vi "SWERVE_MODULE_ACQUIRE.vi"(7 "MC type Drv":T1(ring), 8 "Drv Gear Ratio":dbl, 9 "Wheel Diameter IN":dbl=4.0 format="%#_13g", 10 "Encoder Name":string, 11 "Drive Motor Name":string) -> (0 "SWERVE_DRIVE_MODULE_POSITION":T2={"Distance"=0.0, "Angle"={"VALUE"=0.0, "COS"=1.0, "SIN"=0.0}, "P"=FALSE} {"Angle"."SIN" format="%13.4f"; "Angle"."COS" format="%13.4f"; "Angle"."VALUE" format="%13.4f"}, 2 "SWERVE_DRIVE_MODULE_STATE":T4={"Speed"=0.0, "Angle"={"VALUE"=0.0, "COS"=1.0, "SIN"=0.0}} {"Angle"."SIN" format="%13.4f"; "Angle"."COS" format="%13.4f"; "Angle"."VALUE" format="%13.4f"})   [LabVIEW 2023]
uses:
  <vilib>/Rock Robotics/WPI/ThirdParty/JAS_Junk/TrajLib/Trajectory_Library.lvlib
  <vilib>/Rock Robotics/WPI/ThirdParty/JAS_Junk/TrajLib/TypeDef/DCMOTOR.CTL
  <vilib>/Analysis/Matrix/Datatypes/RealMatrix.ctl
  <vilib>/Analysis/Matrix/NI_Matrix.lvlib
  <vilib>/Rock Robotics/WPI/ThirdParty/JAS_Junk/TrajLib/TypeDef/LINEAR_SYSTEM.ctl
  <vilib>/Rock Robotics/WPI/ThirdParty/JAS_Junk/TrajLib/TypeDef/LINEAR_SYSTEM_SIM.ctl
  <vilib>/Rock Robotics/WPI/ThirdParty/JAS_Junk/TrajLib/TypeDef/DCMOTOR_SIM.ctl
  <vilib>/Rock Robotics/Network Tables/NT Read Variant.vi
  SWERVE_DRIVE_GLOBALS.vi
  <vilib>/Rock Robotics/WPI/ThirdParty/Phoenix-LabVIEW/Motor Controller/Get/CTRE_Phoenix_MotorController_GetSelectedSensorData.vi
  <vilib>/Rock Robotics/WPI/ThirdParty/Phoenix-LabVIEW/CANCoder/Get/CTRE_Phoenix_CANcoder_GetSensorData.vi
  <vilib>/Rock Robotics/WPI/ThirdParty/REV Robotics/REVLib/SubVI/Public/SPARK Get Encoder Status Position.vi
  <vilib>/Rock Robotics/WPI/ThirdParty/Phoenix6/getters/GetPRO_PosAndVel_Velocity.vi
  <vilib>/Rock Robotics/WPI/ThirdParty/Phoenix6/getters/GetPRO_PosAndVel_Position.vi
  <vilib>/Rock Robotics/WPI/ThirdParty/REV Robotics/REVLib/SubVI/Public/SPARK Get Encoder Status Velocity.vi
  <vilib>/Rock Robotics/WPI/ThirdParty/JAS_Junk/TrajLib/TypeDef/ROTATION2D.ctl
  <vilib>/Rock Robotics/WPI/ThirdParty/JAS_Junk/TrajLib/TypeDef/SWERVE_DRIVE_MODULE_STATE.ctl
  <vilib>/Rock Robotics/WPI/ThirdParty/JAS_Junk/TrajLib/TypeDef/SWERVE_DRIVE_MODULE_POSITION.ctl
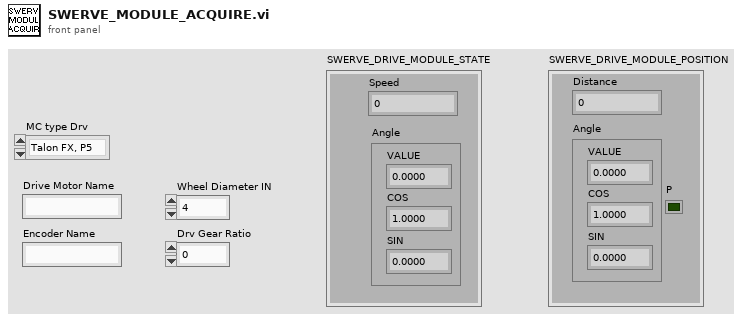
[diagram p1: front panel]
types:
  T1 = enum16{"Talon FX, P5", "Talon FX, P6", "SPARK MAX"}
  T2 = typedef "Trajectory_Library.lvlib/SWERVE_DRIVE_MODULE_POSITION.ctl" = cluster{"Distance":dbl, "Angle":T3, "P":bool}
  T3 = typedef "Trajectory_Library.lvlib/ROTATION2D.ctl" = cluster{"VALUE":dbl, "COS":dbl, "SIN":dbl}
  T4 = typedef "Trajectory_Library.lvlib/SWERVE_DRIVE_MODULE_STATE.ctl" = cluster{"Speed":dbl, "Angle":T3}
  T5 = typedef "Trajectory_Library.lvlib/DCMOTOR_SIM.ctl" = cluster{"LinearSystemSim":T6, "GearBox":T9, "Gearing":dbl}
  T6 = typedef "Trajectory_Library.lvlib/LINEAR_SYSTEM_SIM.ctl" = cluster{"m_Plant":T7, "m_X":T8, "m_Y":T8, "m_U":T8, "MeasureStdDev":T8}
  T7 = typedef "Trajectory_Library.lvlib/LINEAR_SYSTEM.ctl" = cluster{"m_A":T8, "m_B":T8, "m_C":T8, "m_D":T8, "States":i32, "Inputs":i32, "Outputs":i32}
  T8 = typedef "NI_Matrix.lvlib/RealMatrix.ctl" = dbl[][]
  T9 = typedef "Trajectory_Library.lvlib/DCMOTOR.CTL" = cluster{"nominalVoltage_Volts":dbl, "StallTorque_NM":dbl, "StallCurrent_Amps":dbl, "FreeCurrent_Amps":dbl, "FreeSpeed_RadPerSec":dbl, "R_Ohms":dbl, "KvINV_RadPerSecPerVolt":dbl, "Kt_NMPerAmp":dbl, "L_H":dbl, "Jr_KgM2":dbl}
  T10 = typedef "WPI_MotorControlDeviceRef.ctl" = cluster{"DeviceStatus":errorcluster, "Type":T11, "PWM":cluster{"PWM Channel":T12, "DeadBand":T13}, "CAN":cluster{"Device Number":u8, "SetOutput VI Ref":variant, "GetOutput VI Ref":variant, "Enable VI Ref":variant, "Disable VI Ref":variant, "Data":variant}, "Invert":bool, "DIO PWM":cluster{"PWM \"Enable\" Channel":T12, "DIOChannel":T14, "PWM Rate":dbl}}
  T11 = typedef "WPI_MotorControlType.ctl" = enum16{"PWM", "CAN", "DIO PWM"}
  T12 = typedef "FPGA_DIOPWMChannel.ctl" = enum8{"PWM 0", "PWM 1", "PWM 2", "PWM 3", "PWM 4", "PWM 5", "PWM 6", "PWM 7", "PWM 8", "PWM 9", "PWM MXP 0", "PWM MXP 1", "PWM MXP 2", "PWM MXP 3", "PWM MXP 4", "PWM MXP 5", "PWM MXP 6", "PWM MXP 7", "PWM MXP 8", "PWM MXP 9", "Invalid"}
  T13 = typedef "WPI_PWMDeadband.ctl" = cluster{"Name":string, "maxPositivePwm":i32, "minPositivePwm":i32, "centerPwm":i32, "maxNegativePwm":i32, "minNegativePwm":i32, "angularRange":u16}
  T14 = typedef "FPGA_DIOChannel.ctl" = enum8{"DIO 0", "DIO 1", "DIO 2", "DIO 3", "DIO 4", "DIO 5", "DIO 6", "DIO 7", "DIO 8", "DIO 9", "DIO MXP 0", "DIO MXP 1", "DIO MXP 2", "DIO MXP 3", "DIO MXP 4", "DIO MXP 5", "DIO MXP 6", "DIO MXP 7", "DIO MXP 8", "DIO MXP 9", "DIO MXP 10", "DIO MXP 11", "DIO MXP 12", "DIO MXP 13", "DIO MXP 14", "DIO MXP 15", "SPI Port CS1", "SPI Port CS2", "SPI Port CS3", "SPI Port MISO", "SPI Port MOSI", "Invalid"}
  T15 = typedef "DeviceReference.ctl" = cluster{"CANbus Name":string, "Device Encoding":u32, "Device Name":string}
  T16 = cluster{"Value":dbl, "System Timestamp":dbl, "CANivore Timestamp":dbl, "ECU Timestamp":dbl}
  T17 = typedef "CTRE_Phoenix_CANcoder_DeviceRef.ctl" = cluster{"DeviceStatus":errorcluster, "Device Number":u8, "Handle":u64, "UsageFrame":u32, "Library Path":path}
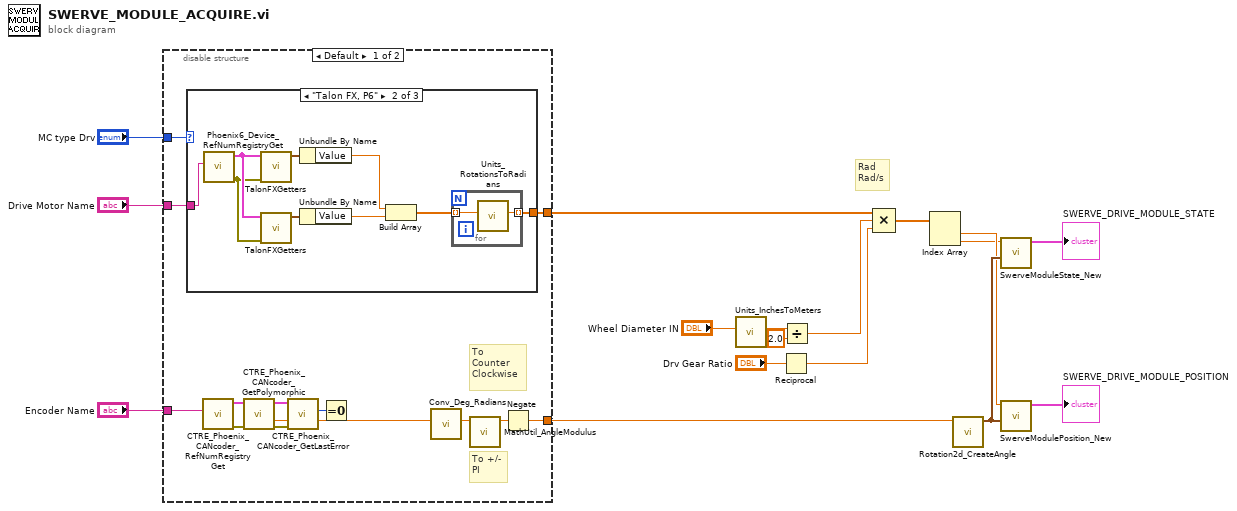
[diagram p0: block diagram]
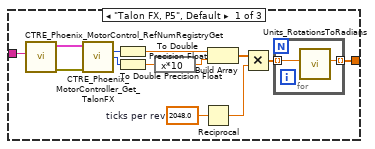
[diagram p2: hidden frame]
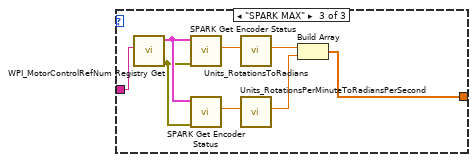
[diagram p3: hidden frame]
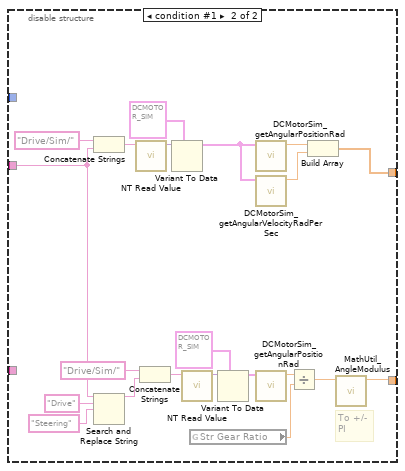
[diagram p4: hidden frame]
diagram:
  # "Rad\nRad/s"
  n1 = disable-structure shown="Default" {
    disable-tunnel: [w27 w78] -> w10
    disable-tunnel: "Drive Motor Name" -> [w23 w65]
    disable-tunnel: "Encoder Name" -> [w22 _]
    disable-tunnel: "MC type Drv" -> [w21 _]
    disable-tunnel: [w18 w69] -> w1
    frame condition #0 (active) {
      # "To\nCounter\nClockwise"
      # "To +/-\nPI"
      n2 = case shown="\"Talon FX, P6\"" w21 {
        tunnel: w23 -> [w38 w53 w64]
        tunnel: [w31 w54 w61] -> w27
        frame "Talon FX, P5", Default {
          w37 = 2048.0  # ticks per rev
          n3 = call <vilib>:"CTRE_Phoenix_MotorControl_RefNumRegistryGet.vi"("refnum name"=w38) -> ("error out"=w39:errorcluster, "PhoenixMotorControlDevRef"=w40:T10)  [unwired: 9 in]
          n4 = call-poly <vilib>:"CTRE_Phoenix_MotorController_Get_TalonFX.vi"("PhoenixMotorControlDevRef"=w40, "error in"=w39) -> ("Position (Raw Sensor Units)"=w43:i32, "Velocity (Raw Sensor Units per 100 ms)"=w41:i32)  [unwired: 10 in, 2 out]
          n5 = To Double Precision Float(number=w43) -> (double precision float=w36:dbl)
          n6 = To Double Precision Float(number=w41) -> (double precision float=w42:dbl)
          n7 = expression code="x*10"(w42) -> (w35:dbl)
          n8 = Reciprocal(x=w37) -> (1/x=w33:dbl)
          n9 = Build Array(w36, w35) -> (w34:dbl[])
          n10 = Multiply(x=w34, y=w33) -> (x*y=w32:dbl[])
          n11 = for {
            tunnel: w32 -> [w45] mode=indexing
            tunnel: [w44] -> w31 mode=indexing
            n12 = call <vilib>:"Units_RotationsToRadians.vi"("Rotations"=w45) -> ("Radians"=w44:dbl)  [unwired: 10 in]
          }
        }
        frame "Talon FX, P6" {
          n13 = call <vilib>:"Phoenix6_Device_RefNumRegistryGet.vi"("refnum name"=w53) -> ("error out"=w51:errorcluster, "data"=w52:T15)  [unwired: 9 in]
          n14 = call-poly <vilib>:"TalonFXGetters.vi"("error in"=w51, "DeviceReference"=w52) -> ("Output"=w49:T16)  [unwired: 8 in, 1 out]
          n15 = call-poly <vilib>:"TalonFXGetters.vi"("error in"=w51, "DeviceReference"=w52) -> ("Output"=w48:T16)  [unwired: 8 in, 1 out]
          n16 = Unbundle By Name(w49) -> ("Value"=w46:dbl)
          n17 = Unbundle By Name(w48) -> ("Value"=w47:dbl)
          n18 = Build Array(w46, w47) -> (w50:dbl[])
          n19 = for {
            tunnel: w50 -> [w56] mode=indexing
            tunnel: [w55] -> w54 mode=indexing
            n20 = call <vilib>:"Units_RotationsToRadians.vi"("Rotations"=w56) -> ("Radians"=w55:dbl)  [unwired: 10 in]
          }
        }
        frame "SPARK MAX" {
          n21 = call <vilib>:"WPI_MotorControlRefNum Registry Get.vi"("refnum name"=w64) -> ("error out"=w57:errorcluster, "MotorControlDevRef"=w58:T10)  [unwired: 9 in]
          n22 = call-poly <vilib>:"SPARK Get Encoder Status.vi"("error in (no error)"=w57, "MotorControlDevRef in"=w58) -> ("Sensor Position"=w59:dbl)  [unwired: 6 in, 3 out]
          n23 = call-poly <vilib>:"SPARK Get Encoder Status.vi"("error in (no error)"=w57, "MotorControlDevRef in"=w58) -> ("Sensor Velocity"=w60:dbl)  [unwired: 6 in, 3 out]
          n24 = call <vilib>:"Units_RotationsToRadians.vi"("Rotations"=w59) -> ("Radians"=w63:dbl)  [unwired: 10 in]
          n25 = call <vilib>:"Units_RotationsPerMinuteToRadiansPerSecond.vi"("RotationsPerMinute"=w60) -> ("RadiansPerSecond"=w62:dbl)  [unwired: 10 in]
          n26 = Build Array(w63, w62) -> (w61:dbl[])
        }
      }
      n27 = call <vilib>:"CTRE_Phoenix_CANcoder_RefNumRegistryGet.vi"("refnum name"=w22) -> ("error out"=w30:errorcluster, "CTRE_CANcoder_DeviceRef"=w29:T17)  [unwired: 9 in]
      n28 = call-poly <vilib>:"CTRE_Phoenix_CANcoder_GetPolymorphic.vi"("CTRE_CANcoder_DeviceRef"=w29, "error in"=w30) -> ("CTRE_CANcoder_DeviceRef"=w26:T17, "Absolute Position"=w28:dbl, "error out"=w25:errorcluster)  [unwired: 9 in, 2 out]
      n29 = call <vilib>:"CTRE_Phoenix_CANcoder_GetLastError.vi"("error in"=w25, "CTRE_CANcoder_DeviceRef"=w26) -> ("Last Error Code"=w24:i8)  [unwired: 7 in, 2 out]
      n30 = Equal To 0?(x=w24) -> ()  [unwired: 1 out]
      n31 = call <vilib>:"Conv_Deg_Radians.vi"("Degress"=w28) -> ("Radians"=w19:dbl)  [unwired: 10 in]
      n32 = call <vilib>:"MathUtil_AngleModulus.vi"("InputAngle"=w19) -> ("ModulsAngle"=w20:dbl)  [unwired: 10 in]
      n33 = Negate(x=w20) -> (-x=w18:dbl)
    }
    frame condition #1 {
      # "To +/-\nPI"
      n34 = Concatenate Strings("Drive/Sim/" ("name"), w65) -> (w83:string)
      n35 = Search and Replace String(input string=w65, search string="Drive" ("substring (\"\")"), replace string="Steering" ("replace string (\"\")")) -> (result string=w66:string)  [unwired: 5 in, 3 out]
      n36 = call-poly <vilib>:"NT Read Value.vi"("name"=w83) -> ("Variant"=w85:variant)  [unwired: 9 in, 1 out]
      n37 = Concatenate Strings("Drive/Sim/" ("name"), w66) -> (w73:string)
      n38 = Variant To Data(type=T5 {"LinearSystemSim"={"m_Plant"={"m_A"=[], "m_B"=[], "m_C"=[], "m_D"=[], "States"=0, "Inputs"=0, "Outputs"=0}, "m_X"=[], "m_Y"=[], "m_U"=[], "MeasureStdDev"=[]}, "GearBox"={"nominalVoltage_Volts"=0.0, "StallTorque_NM"=0.0, "StallCurrent_Amps"=0.0, "FreeCurrent_Amps"=0.0, "FreeSpeed_RadPerSec"=0.0, "R_Ohms"=0.0, "KvINV_RadPerSecPerVolt"=0.0, "Kt_NMPerAmp"=0.0, "L_H"=0.0, "Jr_KgM2"=0.0}, "Gearing"=0.0} ("DCMOTOR_SIM"), Variant=w85) -> (data=w81:T5)  [unwired: 1 in, 1 out]
      n39 = call-poly <vilib>:"NT Read Value.vi"("name"=w73) -> ("Variant"=w72:variant)  [unwired: 9 in, 1 out]
      n40 = global read "SWERVE_DRIVE_GLOBALS.vi" "Str Gear Ratio"() -> (w70:dbl)
      n41 = Variant To Data(type=T5 {"LinearSystemSim"={"m_Plant"={"m_A"=[], "m_B"=[], "m_C"=[], "m_D"=[], "States"=0, "Inputs"=0, "Outputs"=0}, "m_X"=[], "m_Y"=[], "m_U"=[], "MeasureStdDev"=[]}, "GearBox"={"nominalVoltage_Volts"=0.0, "StallTorque_NM"=0.0, "StallCurrent_Amps"=0.0, "FreeCurrent_Amps"=0.0, "FreeSpeed_RadPerSec"=0.0, "R_Ohms"=0.0, "KvINV_RadPerSecPerVolt"=0.0, "Kt_NMPerAmp"=0.0, "L_H"=0.0, "Jr_KgM2"=0.0}, "Gearing"=0.0} ("DCMOTOR_SIM"), Variant=w72) -> (data=w75:T5)  [unwired: 1 in, 1 out]
      n42 = call <vilib>:"DCMotorSim_getAngularPositionRad.vi"("DCMotorSim"=w81) -> ("Position_Rad"=w80:dbl)  [unwired: 10 in]
      n43 = call <vilib>:"DCMotorSim_getAngularVelocityRadPerSec.vi"("DCMotorSim"=w81) -> ("Velocity_RadPerSec"=w79:dbl)  [unwired: 10 in]
      n44 = call <vilib>:"DCMotorSim_getAngularPositionRad.vi"("DCMotorSim"=w75) -> ("Position_Rad"=w71:dbl)  [unwired: 10 in]
      n45 = Divide(x=w71, y=w70) -> (x/y=w68:dbl)
      n46 = Build Array(w80, w79) -> (w78:dbl[])
      n47 = call <vilib>:"MathUtil_AngleModulus.vi"("InputAngle"=w68) -> ("ModulsAngle"=w69:dbl)  [unwired: 10 in]
    }
  }
  n48 = call <vilib>:"Units_InchesToMeters.vi"("Inches"="Wheel Diameter IN") -> ("Meters"=w15:dbl)  [unwired: 10 in]
  n49 = Reciprocal(x="Drv Gear Ratio") -> (1/x=w12:dbl)
  n50 = Divide(x=w15, y=2.0) -> (x/y=w11:dbl)
  n51 = Compound Arithmetic op=MULTIPLY(w10, w11, w12) -> (w9:dbl[])
  n52 = Index Array(array=w9) -> (element #1=w8:dbl, element #2=w2:dbl)  [unwired: 2 in]
  n53 = call <vilib>:"Rotation2d_CreateAngle.vi"("Angle"=w1) -> ("ROTATION"=w16:T3)  [unwired: 10 in]
  n54 = call <vilib>:"SwerveModuleState_New.vi"("ROTATION"=w16, "Speed"=w2) -> ("SWERVE_DRIVE_MODULE_STATE"=→"SWERVE_DRIVE_MODULE_STATE":T4)  [unwired: 9 in]
  n55 = call <vilib>:"SwerveModulePosition_New.vi"("ROTATION"=w16, "Distance"=w8) -> ("SWERVE_DRIVE_MODULE_POSITION"=→"SWERVE_DRIVE_MODULE_POSITION":T2)  [unwired: 9 in]
